vi "PIcontroll.vi"(9 "2.1.3 Steering gains":T1={"proportional gain (Kc)"=1.0, "integral gain (Kc*Ts/Ti)"=1.66796875, "derivative gain (Kc*Td/Ts)"=0.0} {"proportional gain (Kc)" format="%.11g"; "integral gain (Kc*Ts/Ti)" format="%.11g"; "derivative gain (Kc*Td/Ts)" format="%.11g"}, 10 "Setpoint":i32, 11 "Steering Encoder":i32) -> (2 "Output":fxp<+/-,19,4> format="%.21g")   [LabVIEW 2010]
doc: "PID controll for FPGA (fixed point math) without the \"I\" or the \"D\""
uses:
  1.0-Hindbrain Global.vi
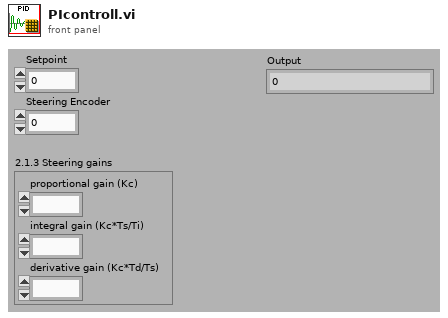
[diagram p1: front panel]
types:
  T1 = cluster{"proportional gain (Kc)":fxp<+/-,16,8>, "integral gain (Kc*Ts/Ti)":fxp<+/-,16,8>, "derivative gain (Kc*Td/Ts)":fxp<+/-,16,8>}
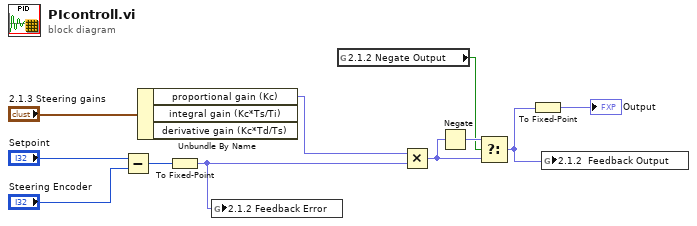
[diagram p0: block diagram]
diagram:
  n1 = Subtract(x="Setpoint", y="Steering Encoder") -> (x-y=w8:i32)
  n2 = Unbundle By Name("2.1.3 Steering gains") -> ("proportional gain (Kc)"=w2:fxp<+/-,16,8>)  [unwired: 2 out]
  n3 = To Fixed-Point(number=w8) -> (fixed-point=w3:fxp<+/-,32,32>)  [unwired: 1 in]
  n4 = global write "1.0-Hindbrain Global.vi" "2.1.2 Feedback Error"(w3) -> ()
  n5 = global read "1.0-Hindbrain Global.vi" "2.1.2 Negate Output"() -> (w4:bool)
  n6 = Multiply(x=w2, y=w3) -> (x*y=w6:fxp<+/-,48,40>)
  n7 = Negate(x=w6) -> (-x=w5:fxp<+/-,47,39>)
  n8 = Select(t=w5, s=w4, f=w6) -> (s? t:f=w7:fxp<+/-,48,40>)
  n9 = To Fixed-Point(number=w7) -> (fixed-point=→"Output":fxp<+/-,19,4>)  [unwired: 1 in]
  n10 = global write "1.0-Hindbrain Global.vi" "2.1.2  Feedback Output"(w7) -> ()
